vi "ErrorMSG_difd.vi"(1 "input":bool) -> (0 "output":bool)   [LabVIEW 2019]
panel:
  out "pre input":bool
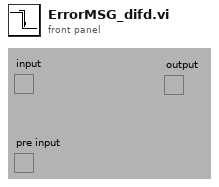
[diagram p1: front panel]
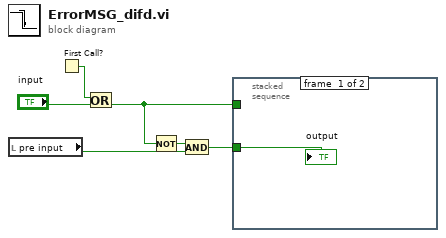
[diagram p0: block diagram]
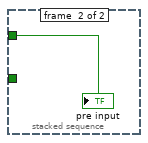
[diagram p2: hidden frame]
diagram:
  n1 = local read "pre input"() -> (w4:bool)
  n2 = First Call?() -> (First Call?: T/F=w1:bool)
  n3 = Or(x=w1, y="input") -> (x .or. y?=w2:bool)
  n4 = Not(x=w2) -> (.not. x?=w5:bool)
  n5 = And(x=w5, y=w4) -> (x .and. y?=w6:bool)
  n6 = stacked-sequence {
    tunnel: w6 -> [w7 _]
    tunnel: w2 -> [_ w8]
    frame #0 {
      "output" <- w7
    }
    frame #1 {
      "pre input" <- w8
    }
  }
